vi "WebSockets Server.vi"() -> ()   [LabVIEW 2020]
uses:
  Type Defs/State.ctl
  <vilib>/ActorFramework/Message Enqueuer/Message Enqueuer.lvclass/Message Enqueuer.ctl
  Libraries/RPI.SenseHat.Actor/RPI.SenseHat.Actor Messages/Fill Display Msg/Fill Display Msg.lvclass/Fill Display Msg.ctl
  Libraries/RPI.SenseHat.Actor/RPI.SenseHat.Actor Messages/Draw Display Msg/Draw Display Msg.lvclass/Draw Display Msg.ctl
  <vilib>/MediaMongrels Ltd/WebSockets/WebSockets/WebSocket Server/WebSocket Server.lvclass
  C:/Program Files (x86)/National Instruments/LabVIEW 2020/vi.lib/MediaMongrels Ltd/WebSockets/WebSockets/WebSocket/WebSocket.lvclass
  <vilib>/MediaMongrels Ltd/WebSockets/Sockets/VISA TCP Listener/VISA TCP Listener.lvclass
  <vilib>/ActorFramework/Message Enqueuer/Enqueue.vi
  Libraries/RPI.SenseHat.Actor/RPI.SenseHat.Actor Messages/Reset Display Msg/Reset Display Msg.lvclass
  C:/Program Files (x86)/National Instruments/LabVIEW 2020/vi.lib/ActorFramework/Message/Message.lvclass
  Libraries/RPI.SenseHat.Actor/RPI.SenseHat.Actor Messages/Clear Display Msg/Clear Display Msg.lvclass
  Libraries/RPI.SenseHat.Actor/RPI.SenseHat.Actor Messages/Fill Display Msg/Fill Display Msg.lvclass
  Libraries/RPI.SenseHat.Actor/RPI.SenseHat.Actor Messages/Draw Display Msg/Draw Display Msg.lvclass
  <vilib>/ActorFramework/Stop Msg/Stop Msg.lvclass
  <vilib>/ActorFramework/Message Priority Queue/Priority Enqueue.vi
  <vilib>/MediaMongrels Ltd/WebSockets/WebSockets/WebSocket/WebSocket.lvclass
  Libraries/RPI.SenseHat.Actor/RPI.SenseHat.Actor.lvlib
  Libraries/RPI.SenseHat.Actor/RPI.SenseHat.Actor Messages/Get Joystick State Msg WFR/Get Joystick State Msg WFR.lvclass
  <vilib>/addons/_JKI.lib/Serialization/JSON/JKI JSON Serialization.lvlib
panel:
  out "value 2":string caption="Current Client Name"
  out "value":string caption="Current tasks"
  out "IP Address":string
  in  "Stop":bool
  out "Current Time":string
  # "TCP Port 6123"
  # "ws://host:port"
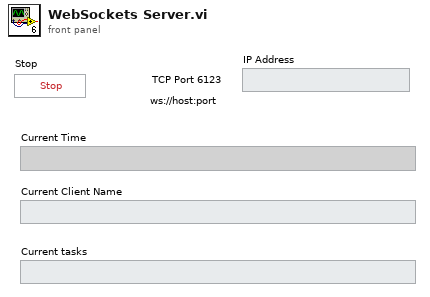
[diagram p1: front panel]
types:
  T1 = typedef "State.ctl" = enum16{"Initialise", "Listen", "Write Data", "Read Data", "Close WebSocket", "Exit"}
  T2 = typedef "RPI.SenseHat.Joystick.lvlib/Joystick.ctl" = cluster{"Enter":bool, "Down":bool, "Up":bool, "Right":bool, "Left":bool}
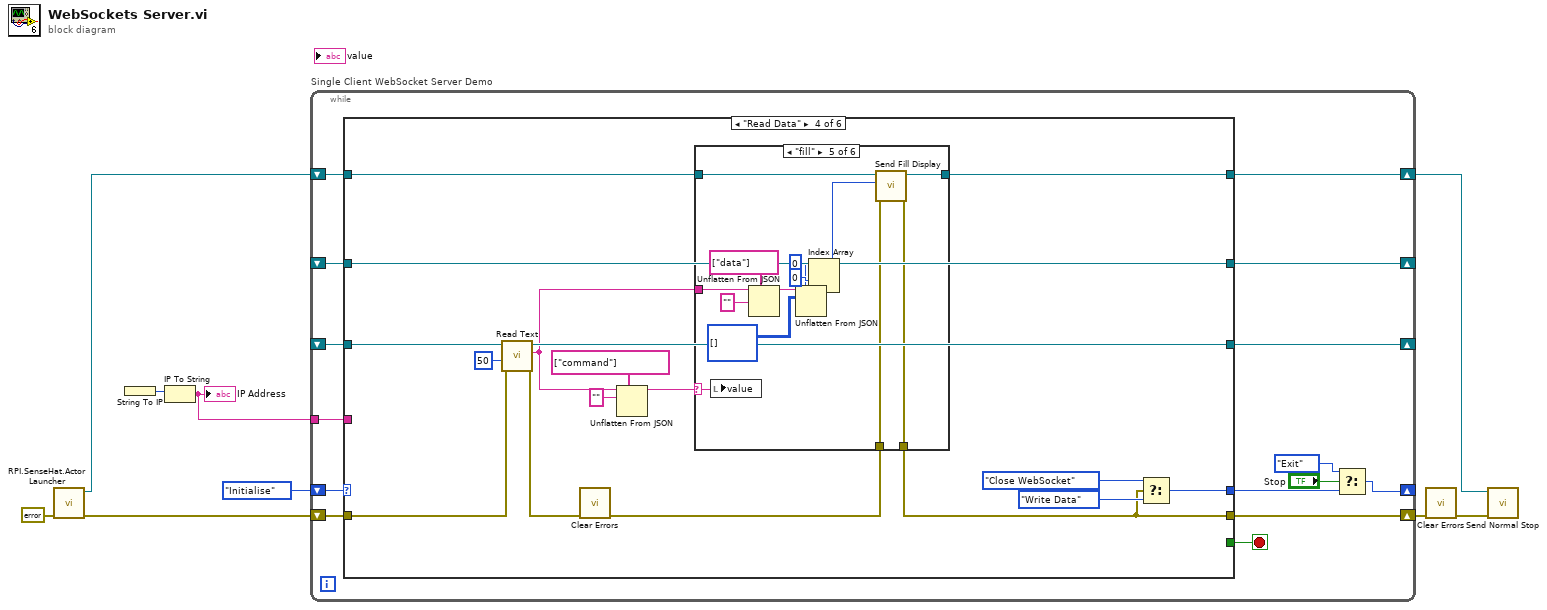
[diagram p0: block diagram]
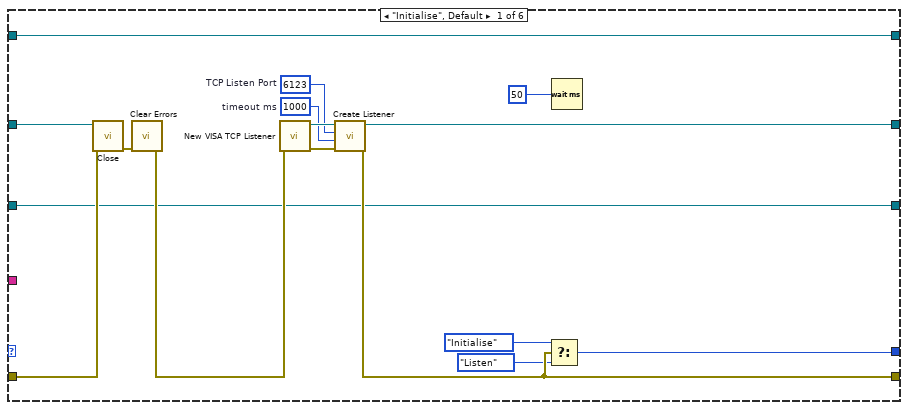
[diagram p2: hidden frame]
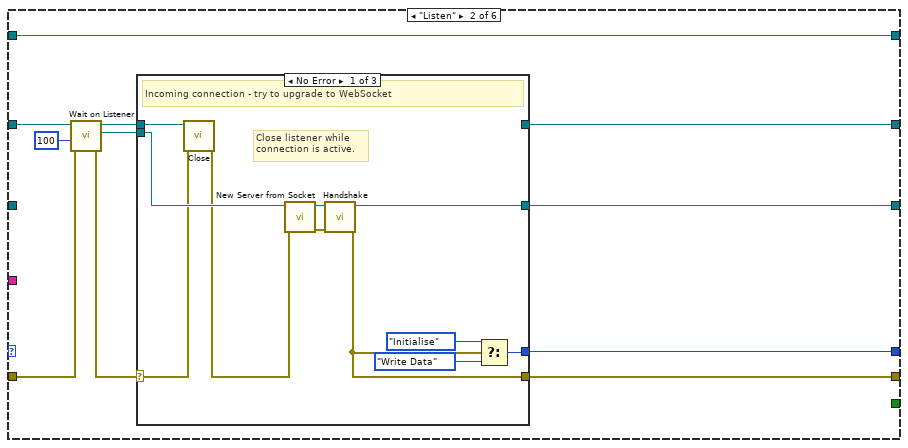
[diagram p3: hidden frame]
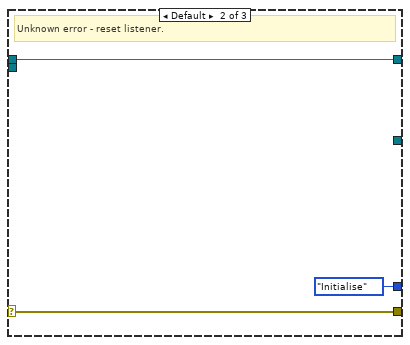
[diagram p4: hidden frame]
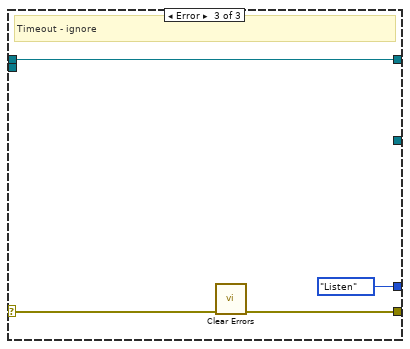
[diagram p5: hidden frame]
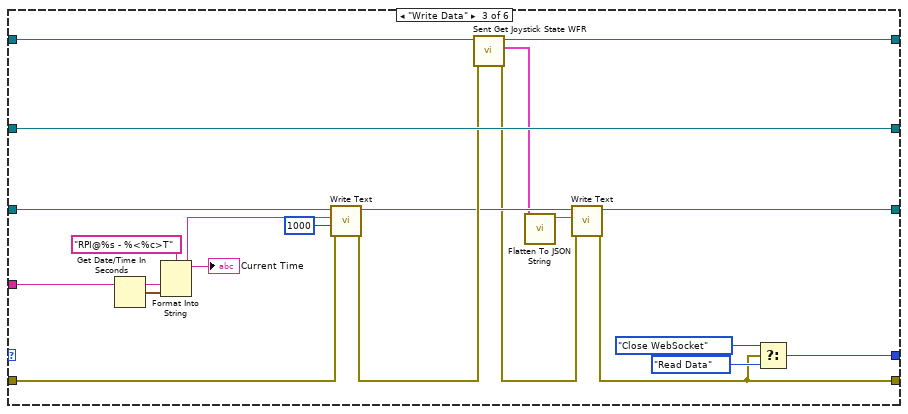
[diagram p6: hidden frame]
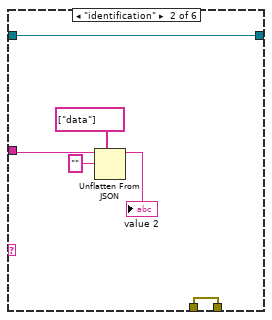
[diagram p8: hidden frame]
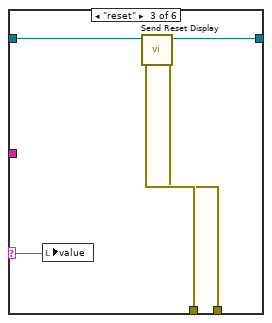
[diagram p9: hidden frame]
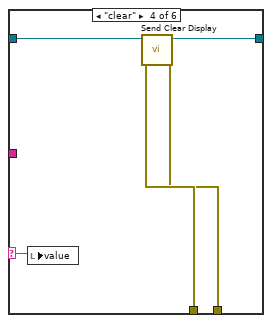
[diagram p10: hidden frame]
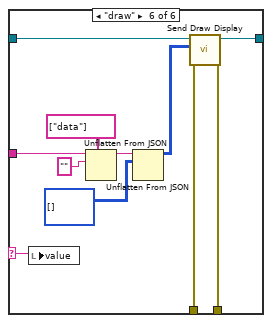
[diagram p11: hidden frame]
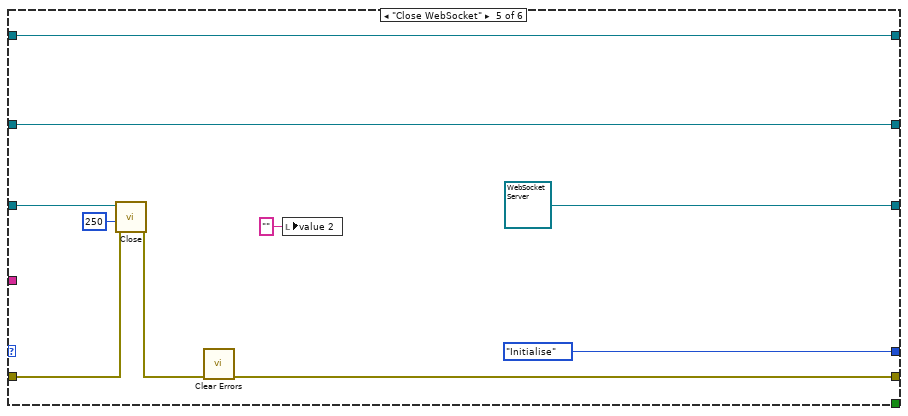
[diagram p12: hidden frame]
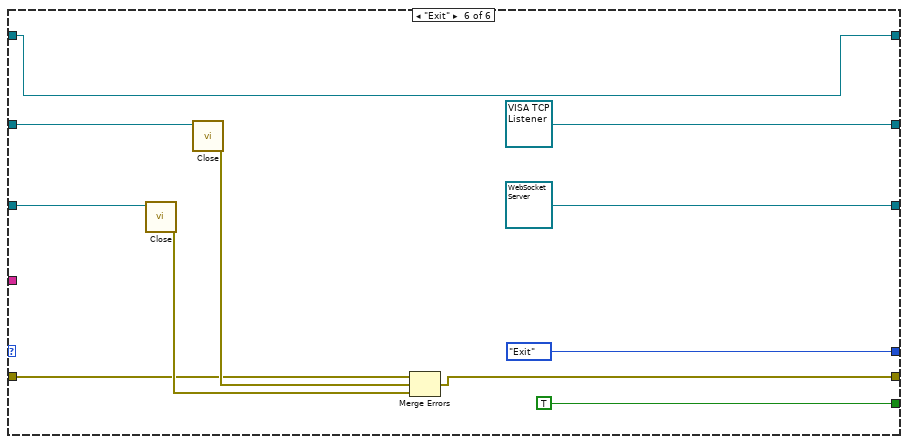
[diagram p13: hidden frame]
diagram:
  n1 = call "RPI.SenseHat.Actor Launcher.vi"("error in (no error)"=errorcluster {"status"=FALSE, "code"=0, "source"=""}) -> ("error out"=w8:errorcluster, "RPI.SenseHat Enqueuer"=w9:refnum<class "Message Enqueuer.lvclass">)  [unwired: 9 in]
  n2 = String To IP() -> (0:w3:u32)  [unwired: 1 in]
  n3 = IP To String(2:w3) -> (0:w1:string)  [unwired: 1 in]
  "IP Address" <- w1
  n4 = while "Single Client WebSocket Server Demo" {
    shift-right: [w13] -> _
    shift-left: State."Initialise" ("Enum") -> [w24]
    shift-right: [w22] -> _
    shift-left: _ -> [w17]
    shift-right: [w21] -> w5
    shift-left: w8 -> [w20]
    shift-right: [w19] -> _
    shift-left: _ -> [w18]
    tunnel: w1 -> [w12]
    shift-right: [w10] -> w2
    shift-left: w9 -> [w11]
    stop <- w23 stop-if-true
    n5 = case shown="\"Read Data\"" w24 {
      tunnel: [_ _ _ _ _ TRUE] -> w23
      tunnel: [w30 w43 w88 w105 State."Initialise" ("Enum") State."Exit" ("Enum")] -> w14
      tunnel: [w34 w46 w89 w106 w152 refnum<class "VISA TCP Listener.lvclass"> refnum ("VISA TCP Listener out")] -> w22
      tunnel: w17 -> [w33 w47 w89 w106 w152 w166]
      tunnel: [w31 w44 w70 w90 w155 w163] -> w21
      tunnel: w20 -> [w32 w45 w82 w94 w156 w164]
      tunnel: [w26 w42 w85 w101 refnum<class "WebSocket Server.lvclass"> refnum ("WebSocket out") refnum<class "WebSocket Server.lvclass"> refnum ("WebSocket out")] -> w19
      tunnel: w18 -> [w26 _ w83 w102 w157 w165]
      tunnel: w12 -> [_ _ w87 _ _ _]
      tunnel: w11 -> [w25 w41 w84 w100 w151 w160]
      tunnel: [w25 w41 w86 w99 w151 w160] -> w10
      frame "Initialise", Default {
        w37 = 1000  # timeout ms
        w38 = u16 6123  # TCP Listen Port
        n6 = call-dynamic "Close.vi"("error in (no error)"=w32, "VISA TCP Listener in"=w33) -> ("error out"=w36:errorcluster)  [unwired: 9 in]
        n7 = call <vilib>:"Clear Errors.vi"("error in (no error)"=w36) -> ("error out"=w35:errorcluster)  [unwired: 5 in, 1 out]
        n8 = call <vilib>:"New VISA TCP Listener.vi"("error in (no error)"=w35) -> ("error out"=w39:errorcluster, "VISA TCP Listener out"=w40:refnum<class "VISA TCP Listener.lvclass">)  [unwired: 9 in]
        n9 = call-dynamic "Create Listener.vi"("error in (no error)"=w39, "timeout ms (5000)"=w37, "Port"=w38, "VISA TCP Listener in"=w40) -> ("error out"=w31:errorcluster, "VISA TCP Listener out"=w34:refnum<class "VISA TCP Listener.lvclass">)  [unwired: 6 in]
        n10 = Select(t=State."Initialise" ("Enum"), s=w31, f=State."Listen" ("Enum")) -> (s? t:f=w30:T1)
        n11 = Wait (ms)(milliseconds to wait=u32 50) -> ()  [unwired: 1 out]
      }
      frame "Listen" {
        n12 = call-dynamic "Wait on Listener.vi"("error in (no error)"=w45, "timeout ms (5000)"=100, "VISA TCP Listener in"=w47) -> ("error out"=w50:errorcluster, "Socket out"=w51:refnum<class "Socket.lvclass">, "VISA TCP Listener out"=w49:refnum<class "VISA TCP Listener.lvclass">)  [unwired: 6 in]
        n13 = case shown="No Error" w50 {
          selector: w50 -> [w58 w65 w69]
          tunnel: w51 -> [w60 _ _]
          tunnel: w49 -> [w57 w64 w68]
          tunnel: [w56 _ _] -> w42
          tunnel: [w55 w65 w66] -> w44
          tunnel: [_ w64 w68] -> w46
          tunnel: [w53 State."Initialise" State."Listen"] -> w43
          frame No Error {
            # "Close listener while connection is active."
            # "Incoming connection - try to upgrade to WebSocket"
            n14 = call-dynamic "Close.vi"("error in (no error)"=w58, "VISA TCP Listener in"=w57) -> ("error out"=w59:errorcluster)  [unwired: 9 in]
            n15 = call <vilib>:"New Server from Socket.vi"("error in (no error)"=w59, "Socket"=w60) -> ("error out"=w61:errorcluster, "WebSocket Server out"=w62:refnum<class "WebSocket Server.lvclass">)  [unwired: 8 in]
            n16 = call-dynamic "Handshake.vi"("error in (no error)"=w61, "WebSocket Connection in"=w62) -> ("error out"=w55:errorcluster, "WebSocket Connection out"=w56:refnum<class "WebSocket Server.lvclass">)  [unwired: 8 in]
            n17 = Select(t=State."Initialise", s=w55, f=State."Write Data") -> (s? t:f=w53:T1)
          }
          frame Default {
            # "Unknown error - reset listener."
          }
          frame Error {
            # "Timeout - ignore"
            n18 = call <vilib>:"Clear Errors.vi"("error in (no error)"=w69) -> ("error out"=w66:errorcluster)  [unwired: 5 in, 1 out]
          }
        }
      }
      frame "Write Data" {
        n19 = Get Date/Time In Seconds() -> (seconds since 1Jan1904=w76:timestamp)
        n20 = Format Into String(format string="RPI@%s - %<%c>T", w87, w76) -> (resulting string=w79:string)  [unwired: 2 in, 1 out]
        "Current Time" <- w79
        n21 = call-dynamic "Write Text.vi"("error in (no error)"=w82, "timeout ms (5000)"=1000, "String Data"=w79, "WebSocket in"=w83) -> ("error out"=w75:errorcluster, "WebSocket out"=w74:refnum<class "WebSocket.lvclass">)  [unwired: 6 in]
        n22 = call "Sent Get Joystick State WFR.vi"("error in (no error)"=w75, "Message Enqueuer"=w84) -> ("error out"=w73:errorcluster, "Reply"=w72:T2, "Message Enqueuer out"=w86:refnum<class "Message Enqueuer.lvclass">)  [unwired: 7 in]
        n23 = call <vilib>:"Flatten To JSON String.vi"("Variant"=w72) -> ("JSON String"=w71:string)  [unwired: 9 in, 1 out]
        n24 = call-dynamic "Write Text.vi"("error in (no error)"=w73, "String Data"=w71, "WebSocket in"=w74) -> ("error out"=w70:errorcluster, "WebSocket out"=w85:refnum<class "WebSocket.lvclass">)  [unwired: 7 in]
        n25 = Select(t=State."Close WebSocket" ("Enum"), s=w70, f=State."Read Data" ("Enum")) -> (s? t:f=w88:T1)
      }
      frame "Read Data" {
        n26 = call-dynamic "Read Text.vi"("error in (no error)"=w94, "timeout ms (5000)"=50, "WebSocket in"=w102) -> ("error out"=w93:errorcluster, "Data"=w98:string, "WebSocket out"=w101:refnum<class "WebSocket.lvclass">)  [unwired: 6 in]
        n27 = call <vilib>:"Clear Errors.vi"("error in (no error)"=w93) -> ("error out"=w91:errorcluster)  [unwired: 5 in, 1 out]
        n28 = Unflatten From JSON(path=string[] ["command"], JSON string=w98, type and defaults="" ("command")) -> (value=w95:string)  [unwired: 4 in, 1 out]
        n29 = case shown="\"fill\"" w95 {
          selector: w95 -> [_ _ w115 w120 w130 w145]
          tunnel: w100 -> [w108 w114 w119 w124 w138 w149]
          tunnel: [w108 w114 w118 w123 w137 w148] -> w99
          tunnel: w98 -> [_ w111 _ _ w136 w140]
          tunnel: w91 -> [w107 w110 w117 w122 w132 w147]
          tunnel: [w107 w110 w116 w121 w131 w146] -> w90
          frame "False", Default {
          }
          frame "identification" {
            n30 = Unflatten From JSON(path=string[] ["data"], JSON string=w111, type and defaults="" ("Color")) -> (value=→"value 2":string)  [unwired: 4 in, 1 out]
          }
          frame "reset" {
            n31 = local write "value"(w115) -> ()
            n32 = call "Send Reset Display.vi"("error in (no error)"=w117, "Message Enqueuer"=w119) -> ("error out"=w116:errorcluster, "Message Enqueuer out"=w118:refnum<class "Message Enqueuer.lvclass">)  [unwired: 8 in]
          }
          frame "clear" {
            n33 = local write "value"(w120) -> ()
            n34 = call "Send Clear Display.vi"("error in (no error)"=w122, "Message Enqueuer"=w124) -> ("error out"=w121:errorcluster, "Message Enqueuer out"=w123:refnum<class "Message Enqueuer.lvclass">)  [unwired: 8 in]
          }
          frame "fill" {
            n35 = local write "value"(w130) -> ()
            n36 = Unflatten From JSON(path=string[] ["data"], JSON string=w136, type and defaults="" ("Color")) -> (value=w133:string)  [unwired: 4 in, 1 out]
            n37 = Unflatten From JSON(JSON string=w133, type and defaults=u32[][] []) -> (value=w129:u32[][])  [unwired: 5 in, 1 out]
            n38 = Index Array(array=w129, index (row)=0, index (col)=0 ("disabled index (col)")) -> (element=w127:u32)
            n39 = call "Send Fill Display.vi"("error in (no error)"=w132, "Color"=w127, "Message Enqueuer"=w138) -> ("error out"=w131:errorcluster, "Message Enqueuer out"=w137:refnum<class "Message Enqueuer.lvclass">)  [unwired: 7 in]
          }
          frame "draw" {
            n40 = local write "value"(w145) -> ()
            n41 = Unflatten From JSON(path=string[] ["data"], JSON string=w140, type and defaults="" ("Color")) -> (value=w144:string)  [unwired: 4 in, 1 out]
            n42 = Unflatten From JSON(JSON string=w144, type and defaults=u32[][] []) -> (value=w139:u32[][])  [unwired: 5 in, 1 out]
            n43 = call "Send Draw Display.vi"("error in (no error)"=w147, "Color"=w139, "Message Enqueuer"=w149) -> ("error out"=w146:errorcluster, "Message Enqueuer out"=w148:refnum<class "Message Enqueuer.lvclass">)  [unwired: 7 in]
          }
        }
        n44 = Select(t=State."Close WebSocket" ("Enum"), s=w90, f=State."Write Data" ("Enum")) -> (s? t:f=w105:T1)
      }
      frame "Close WebSocket" {
        n45 = call-dynamic "Close.vi"("error in (no error)"=w156, "timeout ms (5000)"=250, "WebSocket in"=w157) -> ("error out"=w158:errorcluster)  [unwired: 8 in]
        n46 = call <vilib>:"Clear Errors.vi"("error in (no error)"=w158) -> ("error out"=w155:errorcluster)  [unwired: 5 in, 1 out]
        n47 = local write "value 2"("" ("value 2")) -> ()
      }
      frame "Exit" {
        n48 = call-dynamic "Close.vi"("WebSocket in"=w165) -> ("error out"=w168:errorcluster)  [unwired: 10 in]
        n49 = call-dynamic "Close.vi"("VISA TCP Listener in"=w166) -> ("error out"=w167:errorcluster)  [unwired: 10 in]
        n50 = Merge Errors(w164, w167, w168) -> (w163:errorcluster)
      }
    }
    n51 = Select(t=State."Exit" ("Enum"), s="Stop", f=w14) -> (s? t:f=w13:T1)
  }
  n52 = call <vilib>:"Clear Errors.vi"("error in (no error)"=w5) -> ("error out"=w4:errorcluster)  [unwired: 5 in, 1 out]
  n53 = call <vilib>:"Send Normal Stop.vi"("error in (no error)"=w4, "Message Enqueuer"=w2) -> ()  [unwired: 9 in, 1 out]
